vi "Vi scripting temp.vi"   [LabVIEW 2015]
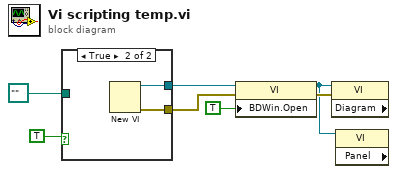
[diagram p0: block diagram]
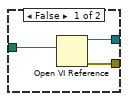
[diagram p2: hidden frame]
diagram:
  n1 = case shown="True" TRUE {
    tunnel: [w9 w12] -> w6
    tunnel: [w8 w11] -> w5
    tunnel: path "" ("vi path") -> [w10 _]
    frame False {
      n2 = Open VI Reference(vi path=w10) -> (vi reference=w9:refnum<vi>, error out=w8:errorcluster)  [unwired: 5 in]
    }
    frame True {
      n3 = New VI() -> (0:w11:errorcluster, 3:w12:refnum<vi>)  [unwired: 7 in]
    }
  }
  n4 = property class="VI"(reference=w6, error in=w5, "BDWin.Open"=TRUE ("Block Diagram Window:Open")) -> (reference out=w3:refnum<vi>, error out=w7:errorcluster)
  n5 = property class="VI" props=["Diagram"](reference=w3, error in=w7) -> ()  [unwired: 3 out]
  n6 = property class="VI" props=["Panel"](reference=w3) -> ()  [unwired: 1 in, 3 out]
